vi "Lockin.DAQ.ErrorHandler.vi"(8 "error in (no error)":errorcluster, 11 "Lockin.DAQ in":refnum<class "Lockin.DAQ.lvclass">) -> (0 "error out":errorcluster, 1 "Error Filtered?":bool, 2 "Filtered Error Details":T1, 3 "Lockin.DAQ out":refnum<class "Lockin.DAQ.lvclass">)   [LabVIEW 2016, in "Lockin.DAQ.lvclass"]
uses:
  Lockin.DAQ.lvclass
  <userlib>/_OpenG.lib/error/error.llb/Filtered Error Details - Cluster__ogtk.ctl
  <userlib>/_OpenG.lib/error/error.llb/Filter Error Codes (Array)__ogtk.vi
  <userlib>/LevyLab/Levylab Instruments/SMOs/Logger.Error/Logger.Error.lvclass
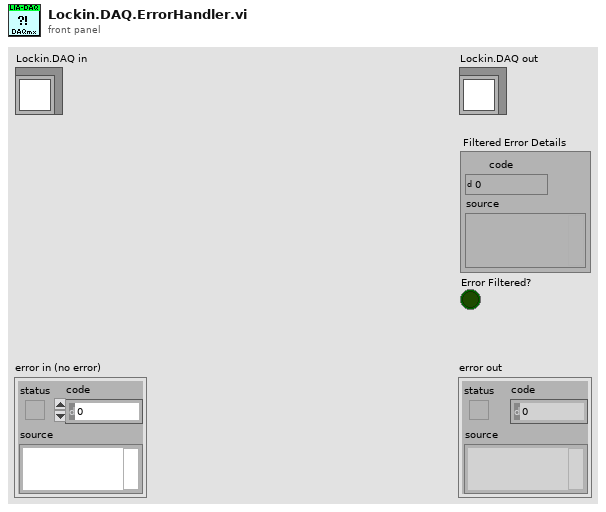
[diagram p1: front panel]
types:
  T1 = typedef "Filtered Error Details - Cluster__ogtk.ctl" = cluster{"code":i32, "source":string}
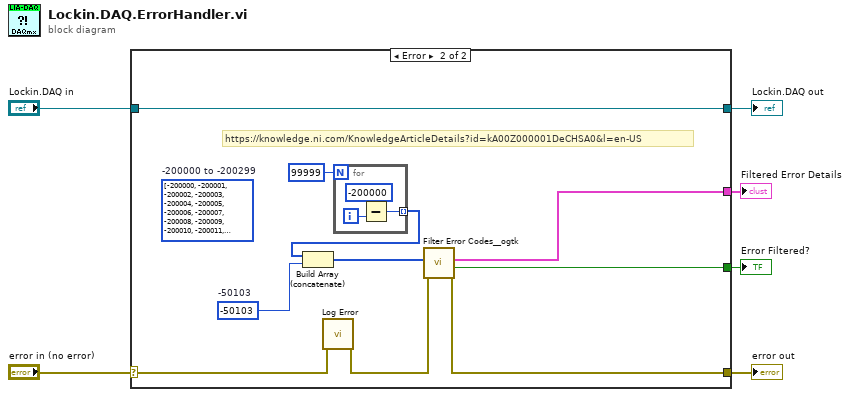
[diagram p0: block diagram]
diagram:
  n1 = case shown="Error" "error in (no error)" {
    selector: "error in (no error)" -> [w7 w12]
    tunnel: [w7 w17] -> w5
    tunnel: [w8 w18] -> w3
    tunnel: "Lockin.DAQ in" -> [w8 w18]
    tunnel: [_ w14] -> w1
    tunnel: [_ w13] -> w2
    frame No Error {
      # "Wire the error cluster across even in the \"No Error\"\ncase so that warnings get propagated."
    }
    frame Error {
      w16 = -50103  # -50103
      (unwired) i32[] [-200000, -200001, -200002, -200003, -200004, -200005, -200006, -200007, -200008, -200009, -200010, -200011, -200012, -200013, -200014, -200015, -200016, -200017, -200018, -200019, -200020, -200021, -200022, -200023, -200024, -200025, -200026, -200027, -200028, -200029, -200030, -200031, -200032, -200033, -200034, -200035, -200036, -200037, -200038, -200039, -200040, -200041, -200042, -200043, -200044, -200045, -200046, -200047, -200048, -200049, -200050, -200051, -200052, -200053, -200054, -200055, -200056, -200057, -200058, -200059, -200060, -200061, -200062, -200063, -200064, -200065, -200066, -200067, -200068, -200069, -200070, -200071, -200072, -200073, -200074, -200075, -200076, -200077, -200078, -200079, -200080, -200081, -200082, -200083, -200084, -200085, -200086, -200087, -200088, -200089, -200090, -200091, -200092, -200093, -200094, -200095, -200096, -200097, -200098, -200099, -200100, -200101, -200102, -200103, -200104, -200105, -200106, -200107, -200108, -200109, -200110, -200111, -200112, -200113, -200114, -200115, -200116, -200117, -200118, -200119, -200120, -200121, -200122, -200123, -200124, -200125, -200126, -200127, -200128, -200129, -200130, -200131, -200132, -200133, -200134, -200135, -200136, -200137, -200138, -200139, -200140, -200141, -200142, -200143, -200144, -200145, -200146, -200147, -200148, -200149, -200150, -200151, -200152, -200153, -200154, -200155, -200156, -200157, -200158, -200159, -200160, -200161, -200162, -200163, -200164, -200165, -200166, -200167, -200168, -200169, -200170, -200171, -200172, -200173, -200174, -200175, -200176, -200177, -200178, -200179, -200180, -200181, -200182, -200183, -200184, -200185, -200186, -200187, -200188, -200189, -200190, -200191, -200192, -200193, -200194, -200195, -200196, -200197, -200198, -200199, -200200, -200201, -200202, -200203, -200204, -200205, -200206, -200207, -200208, -200209, -200210, -200211, -200212, -200213, -200214, -200215, -200216, -200217, -200218, -200219, -200220, -200221, -200222, -200223, -200224, -200225, -200226, -200227, -200228, -200229, -200230, -200231, -200232, -200233, -200234, -200235, -200236, -200237, -200238, -200239, -200240, -200241, -200242, -200243, -200244, -200245, -200246, -200247, -200248, -200249, -200250, -200251, -200252, -200253, -200254, -200255, -200256, -200257, -200258, -200259, -200260, -200261, -200262, -200263, -200264, -200265, -200266, -200267, -200268, -200269, -200270, -200271, -200272, -200273, -200274, -200275, -200276, -200277, -200278, -200279, -200280, -200281, -200282, -200283, -200284, -200285, -200286, -200287, -200288, -200289, -200290, -200291, -200292, -200293, -200294, -200295, -200296, -200297, -200298, -200299]  # -200000 to -200299
      # "https://knowledge.ni.com/KnowledgeArticleDetails?id=kA00Z000001DeCHSA0&l=en-US"
      n2 = call <userlib>:"Log Error.vi"("error in (no error)"=w12) -> ("error out"=w11:errorcluster)  [unwired: 9 in, 1 out]
      n3 = for {
        N: 99999 -> [_]
        tunnel: [w19] -> w9 mode=indexing
        i -> [w21]
        n4 = Subtract(x=-200000, y=w21) -> (x-y=w19:i32)
      }
      n5 = Build Array (concatenate)(w9, w16) -> (w15:i32[])
      n6 = call-poly <userlib>:"Filter Error Codes__ogtk.vi"("Error In"=w11, "Error Codes to Filter"=w15) -> ("Error Out"=w17:errorcluster, "Error Filtered?"=w14:bool, "Filtered Error Details"=w13:T1)  [unwired: 7 in]
    }
  }
  "error out" <- w5
  "Lockin.DAQ out" <- w3
  "Filtered Error Details" <- w2
  "Error Filtered?" <- w1
